vi "OpenConnection_Control1.vi"(8 "error in (no error)":errorcluster, 9 "type":T1, 10 "topicName":string) -> (0 "error out":errorcluster, 3 "reference":refnum<vi>)   [LabVIEW 2012]
uses:
  Typedefs/Control 1.ctl
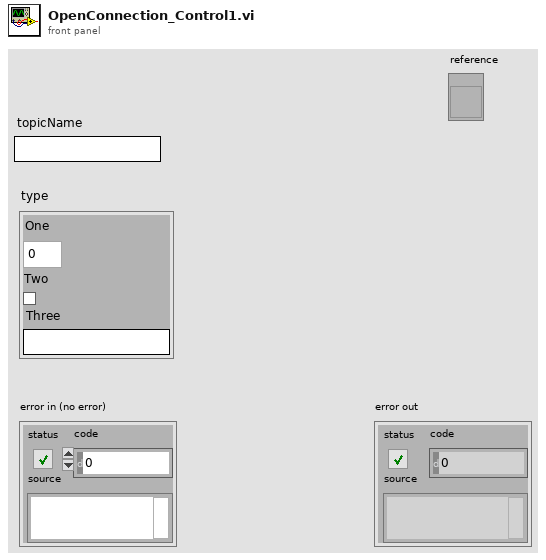
[diagram p1: front panel]
types:
  T1 = typedef "Control 1.ctl" = cluster{"One":dbl, "Two":bool, "Three":string}
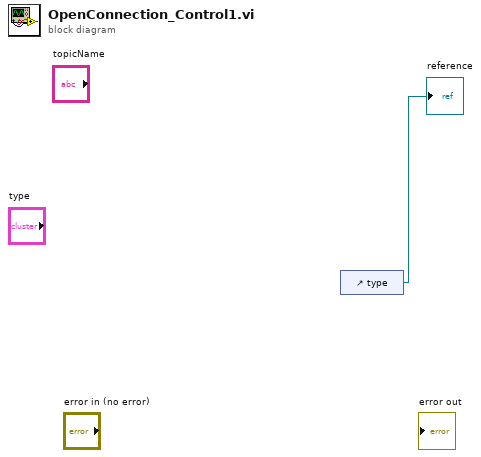
[diagram p0: block diagram]
diagram:
  n1 = control-ref of="type"() -> (→"reference":refnum<vi>)
